vi "LVTracker.vi"(4 "error in":errorcluster, 6 "settings":T2={"Rmax (pix)"=50, "RminZ (pix)"=5, "angular pixel\n coverage factor"=0.7, "radial pixel\n coverage factor"=3.0}, 7 "image in":u8[][](array[numeric])) -> (0 "error in 2":errorcluster)   [LabVIEW 2011]
panel:
  out "position":T1
  out "LV tracker rad prof":dbl[](graph)
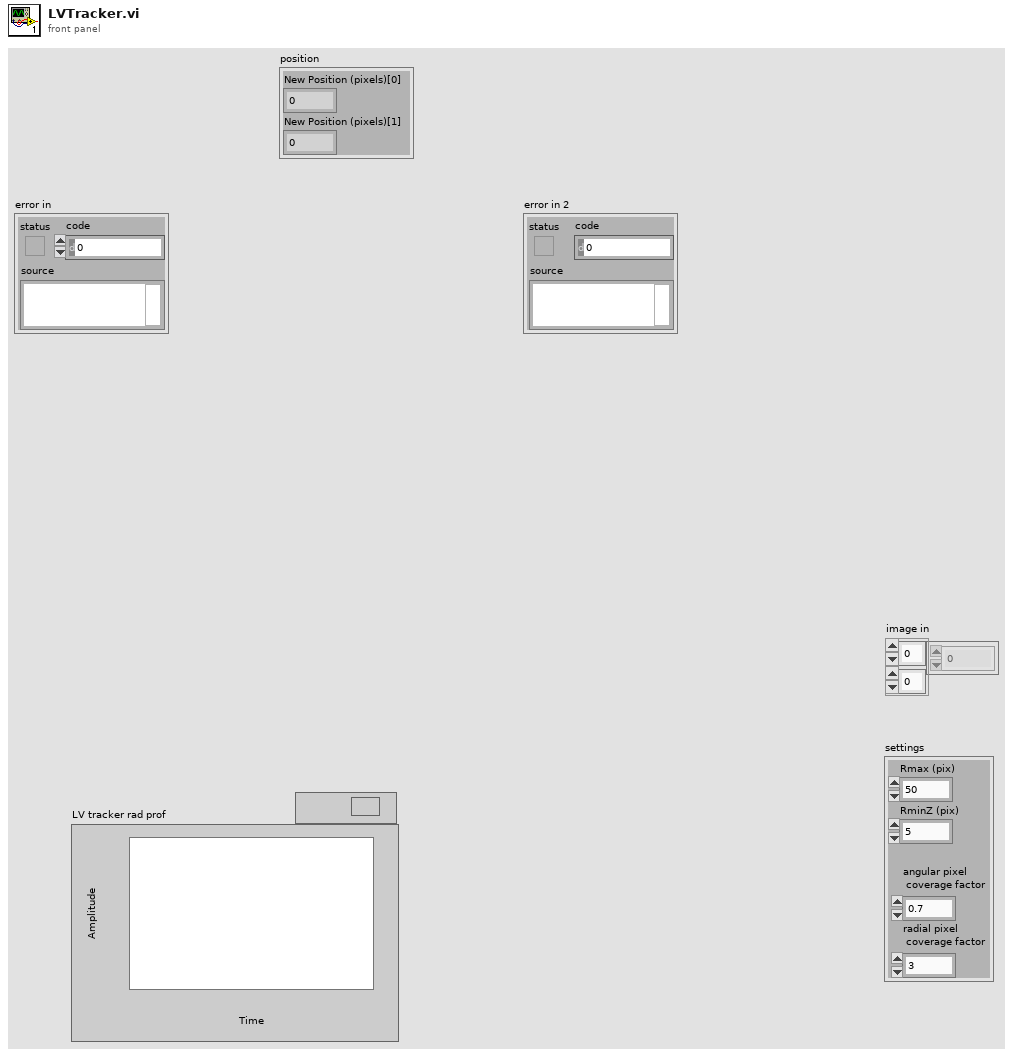
[diagram p1: front panel]
types:
  T1 = cluster{"New Position (pixels)[0]":dbl, "New Position (pixels)[1]":dbl}
  T2 = cluster{"Rmax (pix)":i32, "RminZ (pix)":i32, "angular pixel\n coverage factor":dbl, "radial pixel\n coverage factor":dbl}
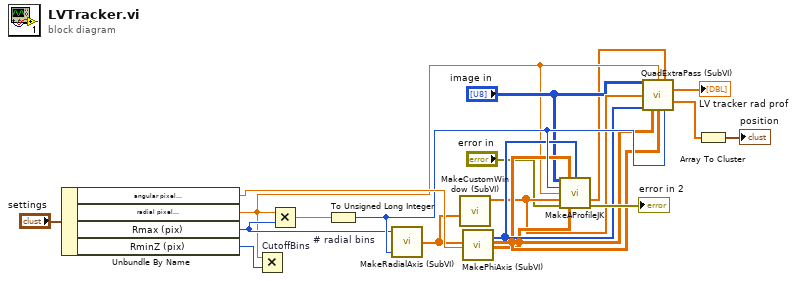
[diagram p0: block diagram]
diagram:
  n1 = Unbundle By Name("settings") -> ("angular pixel\n coverage factor"=w18:dbl, "radial pixel\n coverage factor"=w6:dbl, "Rmax (pix)"=w9:i32, "RminZ (pix)"=w11:i32)
  n2 = Multiply "CutoffBins"(x=w6, y=w11) -> ()  [unwired: 1 out]
  n3 = Multiply(x=w6, y=w9) -> (x*y=w17:dbl)
  n4 = To Unsigned Long Integer "# radial bins"(number=w17) -> (unsigned 32bit integer=w15:u32)
  n5 = call "MakeRadialAxis (SubVI).vi"("# radial bins"=w15, "Rmax-Rmin"=w9) -> ("radialaxis"=w16:dbl[])  [unwired: 1 in]
  n6 = call "MakeCustomWindow (SubVI).vi"("radialaxis"=w16) -> ("Halfstetson"=w10:dbl[])  [unwired: 8 in, 2 out]
  n7 = call "MakePhiAxis (SubVI).vi"("radialBinAxis"=w16, "angular pixel \ncoverage factor"=w18) -> ("lengths"=w14:i32[], "Rsin(phi)[Q]"=w13:dbl[][][], "Rcos(phi)[Q]"=w12:dbl[][][])  [unwired: 2 in, 13 out]
  n8 = call "MakeAProfileJK.vi"("image in"="image in", "Rsin(phi)[Q]"=w13, "angularbinlengths"=w14, "# Radial bins"=w15, "radial bins/pixel"=w6, "window"=w10, "error in (no error) 2"="error in", "Rcos(phi)[Q]"=w12) -> ("xy-out 1"=w5:dbl[], "error in (no error) 3"=→"error in 2":errorcluster)  [unwired: 3 in, 3 out]
  n9 = call "QuadExtraPass (SubVI).vi"("Image"="image in", "radial bins/pixel"=w6, "First position"=w5, "window"=w10, "angularbinlengths"=w14, "Rcos(phi)[Q]"=w12, "Rsin(phi)[Q]"=w13, "# Radial bins"=w15) -> ("radial profile"=→"LV tracker rad prof":dbl[], "New Position (pixels)"=w2:dbl[])  [unwired: 4 in, 2 out]
  n10 = Array To Cluster(array=w2) -> (cluster=→"position":T1)
